vi "upload.list_parts.vi"(8 "error in":errorcluster, 9 "Key":string, 10 "Upload ID":string, 11 "Nominal Client in":refnum<class "Nominal Client.lvclass">) -> (0 "error out":errorcluster, 2 "Parts":T1(array[cluster]), 3 "Nominal Client out":refnum<class "Nominal Client.lvclass">)   [LabVIEW 2020, in "Nominal Client.lvclass"]
doc: "Lists the parts that have been uploaded for a given uploadId."
uses:
  Nominal Client.lvclass
  72e5dcd8-64cf-4027-aada-cf32ea863567.vi
  <vilib>/JDP Science/JSONtext/JSON text to Variant.vi
  <vilib>/JDP Science/JSONtext/LVClass Serializer/JSONtext LVClass Serializer.lvclass
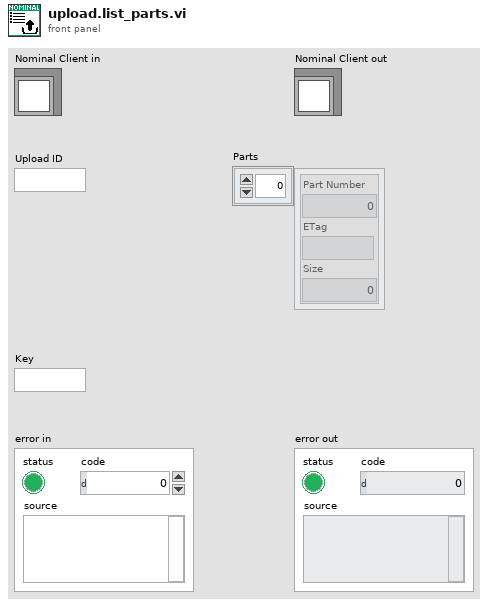
[diagram p1: front panel]
types:
  T1 = cluster{"Part Number":i32, "ETag":string, "Size":i32}[]
  T2 = cluster{"partNumber":i32, "etag":string, "size":i32}[]
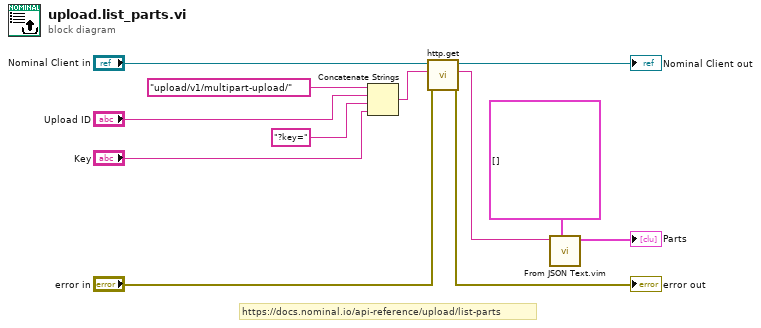
[diagram p0: block diagram]
diagram:
  # "https://docs.nominal.io/api-reference/upload/list-parts"
  n1 = Concatenate Strings("upload/v1/multipart-upload/", "Upload ID", "?key=", "Key") -> (w4:string)
  n2 = call "http.get.vi"("error in"="error in", "Path"=w4, "Nominal Client in"="Nominal Client in") -> ("error out"=→"error out":errorcluster, "Response"=w2:string, "Nominal Client out"=→"Nominal Client out":refnum<class "Nominal Client.lvclass">)  [unwired: 5 in, 1 out]
  n3 = call "From JSON Text.vim"("Data Type and Default Value"=T2 [], "JSON"=w2) -> ("Data out"=→"Parts":T2)  [unwired: 8 in, 1 out]
